vi "Save Difference To File.vi"(2 "save":bool, 4 "path":path, 5 "right":dbl[](array[numeric]), 6 "left":dbl[](array[numeric]), 7 "iteration":dbl[](array[numeric])) -> ()   [LabVIEW 2014]
uses:
  <vilib>/Utility/file.llb/Write To Spreadsheet File (DBL).vi
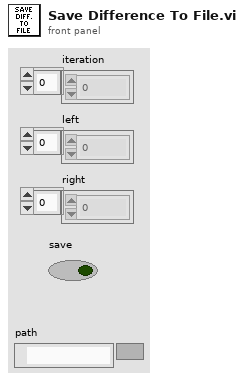
[diagram p1: front panel]
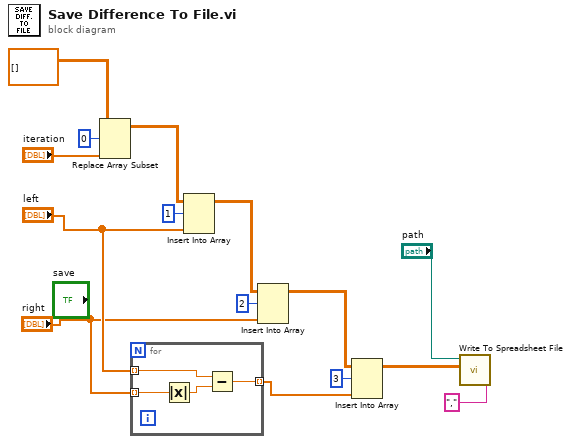
[diagram p0: block diagram]
diagram:
  n1 = Replace Array Subset(array=dbl[][] [], new element="iteration", index (row)=0) -> (w10:dbl[][])  [unwired: 1 in]
  n2 = for {
    tunnel: "left" -> [w19] mode=indexing
    tunnel: "right" -> [w16] mode=indexing
    tunnel: [w18] -> w3 mode=indexing
    n3 = Absolute Value(x=w16) -> (abs(x)=w17:dbl)
    n4 = Subtract(x=w19, y=w17) -> (x-y=w18:dbl)
  }
  n5 = Insert Into Array(array=w10, index (row)=1, new element="left") -> (w8:dbl[][])  [unwired: 1 in]
  n6 = Insert Into Array(array=w8, index (row)=2, new element="right") -> (w6:dbl[][])  [unwired: 1 in]
  n7 = Insert Into Array(array=w6, index (row)=3, new element=w3) -> (w1:dbl[][])  [unwired: 1 in]
  n8 = call-poly <vilib>:"Write To Spreadsheet File.vi"("delimiter (\\t)"="," ("delimiter (\\t)"), "2D data"=w1, "file path (dialog if empty)"="path") -> ()  [unwired: 5 in, 1 out]
